vi "write_params.vi"(8 "error in (no error)":errorcluster caption="entrée d'erreur (pas d'erreur)", 10 "params":T1={"n_iter"=300.0, "tol"=0.001, "alpha_1"=1e-06, "alpha_2"=1e-06, "lambda_1"=1e-06, "lambda_2"=0.0, "compute_score"=FALSE, "threshold_lambda"=10000.0, "fit_intercept"=TRUE, "normalize"=FALSE, "copy_X"=FALSE, "verbose"=FALSE}, 11 "ARDRegression en entrée":refnum<class "ARDRegression.lvclass">) -> (0 "error out":errorcluster caption="sortie d'erreur", 3 "ARDRegression en sortie":refnum<class "ARDRegression.lvclass">)   [LabVIEW 2020, in "ARDRegression.lvclass"]
uses:
  ARDRegression.lvclass
  Controls/ardregressor_params.ctl
  ARDRegression.lvclass/ARDRegression.ctl
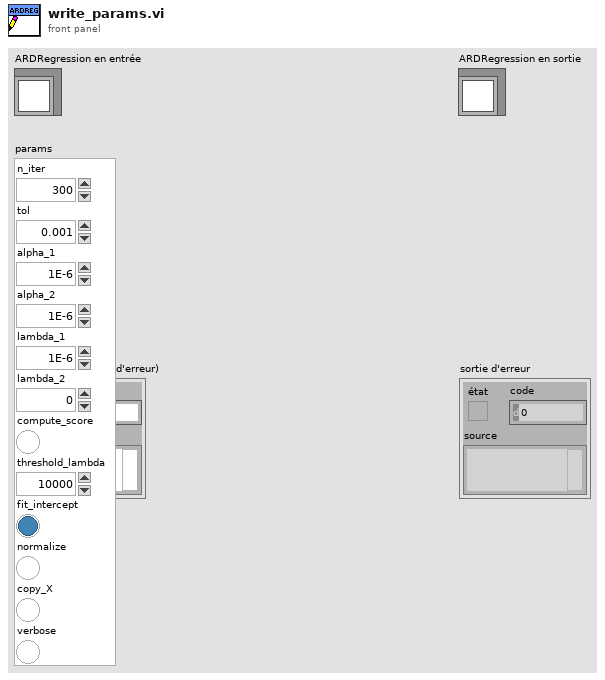
[diagram p1: front panel]
types:
  T1 = typedef "ardregressor_params.ctl" = cluster{"n_iter":dbl, "tol":dbl, "alpha_1":dbl, "alpha_2":dbl, "lambda_1":dbl, "lambda_2":dbl, "compute_score":bool, "threshold_lambda":dbl, "fit_intercept":bool, "normalize":bool, "copy_X":bool, "verbose":bool}
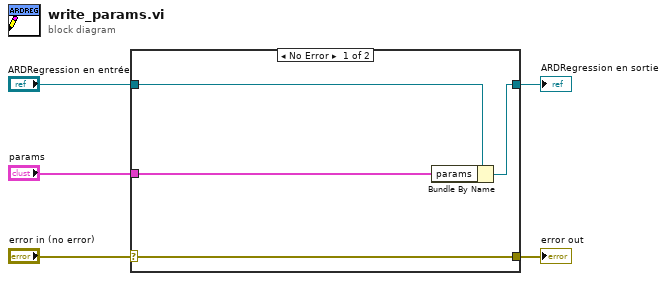
[diagram p0: block diagram]
diagram:
  n1 = case shown="No Error" "error in (no error)" {
    selector: "error in (no error)" -> [w9 w10]
    tunnel: [w9 w10] -> w4
    tunnel: [w7 w11] -> w2
    tunnel: "ARDRegression en entrée" -> [w8 w11]
    tunnel: "params" -> [w6 _]
    frame No Error {
      n2 = Bundle By Name(cluster=w8, "params"=w6) -> (w7:refnum<class "ARDRegression.lvclass">)
    }
    frame Error {
    }
  }
  "error out" <- w4
  "ARDRegression en sortie" <- w2
